vi "Basic Generate LV Icon Template Layer.vi"(8 "error in (no error)":errorcluster) -> (0 "error out":errorcluster, 2 "Picture":picture, 3 "Icon.lvlclass out":refnum<class "Icon.lvclass">)   [LabVIEW 2020, in "LabVIEW Icon API.lvlib"]
doc: "Basic example that shows how to set the Template Layer."
uses:
  LabVIEW Icon API.lvlib
  lv_icon/Classes/Icon/Icon.lvclass
  API_Text.ctl
  <vilib>/picture/picture.llb/imagedata.ctl
  <vilib>/Utility/miscctls.llb/LVPoint32TypeDef.ctl
  API_User Layer Data.ctl
  lv_icon/lv_icon.lvlib
  lv_icon/Controls/Pathes.ctl
panel:
  in  "Layer name":string="Circle"
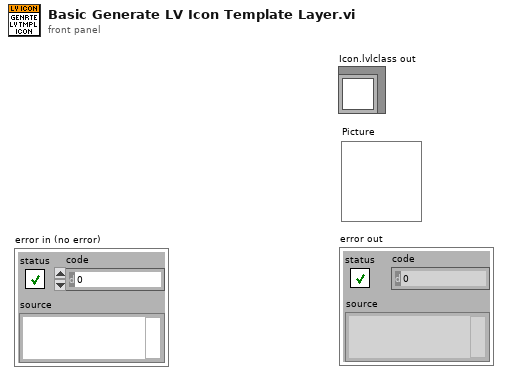
[diagram p1: front panel]
types:
  T1 = typedef "Pathes.ctl" = enum16{"Root Path", "Icon Templates", "Icon Templates VI", "Icon Templates Lib", "Glyphs"}
  T2 = cluster{"left":i16, "top":i16, "right":i16, "bottom":i16}
  T3 = typedef "LabVIEW Icon API.lvlib/API_User Layer Data.ctl" = cluster{"Layer name":string, "Origin":T4, "Icon image data":T5}
  T4 = typedef "LVPoint32TypeDef.ctl" = cluster{"Horizontal":i32, "Vertical":i32}
  T5 = typedef "imagedata.ctl" = cluster{"image type":i32, "image depth":i32, "image":u8[], "mask":u8[], "colors":u32[], "Rectangle":cluster{"left":i16, "top":i16, "right":i16, "bottom":i16}}
  T6 = typedef "LabVIEW Icon API.lvlib/API_Text.ctl" = cluster{"Line 1 text":string, "Line 2 text":string, "Line 3 text":string, "Line 4 text":string}
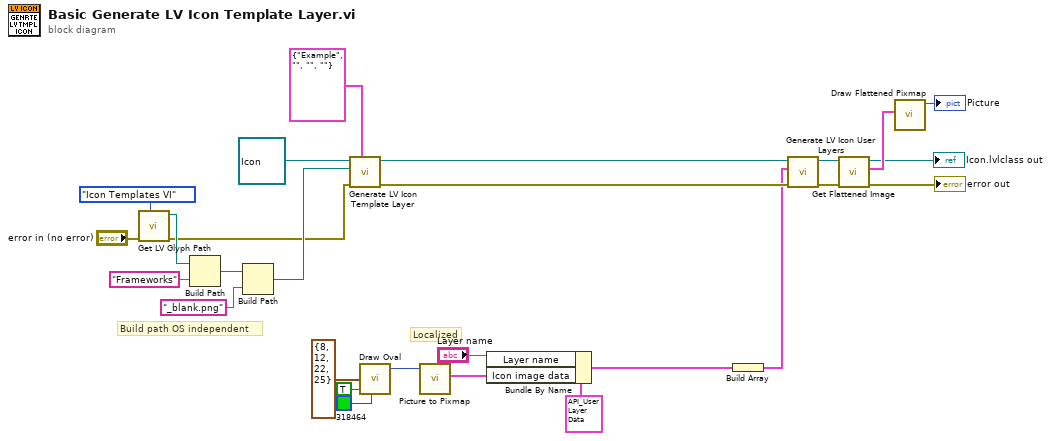
[diagram p0: block diagram]
diagram:
  # "Build path OS independent"
  # "Localized"
  n1 = call "Get LV Glyph Path.vi"("Path"=Pathes."Icon Templates VI", "error in (no error)"="error in (no error)") -> ("error out"=w1:errorcluster, "Requested Path"=w6:path)  [unwired: 1 in, 7 out]
  n2 = Build Path(base path=w6, name or relative path="Frameworks") -> (appended path=w4:path)
  n3 = Build Path(base path=w4, name or relative path="_blank.png") -> (appended path=w2:path)
  n4 = call "Generate LV Icon Template Layer.vi"("Text"=T6 {"Line 1 text"="Example", "Line 2 text"="", "Line 3 text"="", "Line 4 text"=""}, "error in (no error)"=w1, "Template path"=w2, "Icon.lvclass in"=refnum<class "Icon.lvclass"> refnum) -> ("error out"=w24:errorcluster, "Icon.lvclass out"=w23:refnum<class "Icon.lvclass">)  [unwired: 6 in]
  n5 = call <vilib>:"Draw Oval.vi"("rect"=T2 {"left"=8, "top"=12, "right"=22, "bottom"=25}, "fill?(F)"=TRUE, "color(black)"=u32 318464) -> ("new picture"=w17:picture)  [unwired: 6 in]
  n6 = call <vilib>:"Picture to Pixmap.vi"("picture"=w17) -> ("image data"=w15:T5)  [unwired: 9 in, 1 out]
  n7 = Bundle By Name(cluster=T3 {"Layer name"="", "Origin"={"Horizontal"=0, "Vertical"=0}, "Icon image data"={"image type"=0, "image depth"=0, "image"=[], "mask"=[], "colors"=[], "Rectangle"={"left"=0, "top"=0, "right"=0, "bottom"=0}}} ("User layer"), "Layer name"="Layer name", "Icon image data"=w15) -> (w12:T3)
  n8 = Build Array(w12) -> (w11:T3[])
  n9 = call "Generate LV Icon User Layers.vi"("error in (no error)"=w24, "User layers"=w11, "Icon in"=w23) -> ("error out"=w22:errorcluster, "Icon out"=w13:refnum<class "Icon.lvclass">)  [unwired: 7 in]
  n10 = call "Get Flattened Image.vi"("error in (no error)"=w22, "lv_icon.lvlib:Icon.lvclass in"=w13) -> ("error out"=→"error out":errorcluster, "Color Image"=w25:T5, "lv_icon.lvlib:Icon.lvclass out"=→"Icon.lvlclass out":refnum<class "Icon.lvclass">)  [unwired: 6 in, 1 out]
  n11 = call <vilib>:"Draw Flattened Pixmap.vi"("image data"=w25) -> ("new picture"=→"Picture":picture)  [unwired: 8 in]
